vi "Read Summary.vi"(8 "error in (no error)":errorcluster, 11 "WfmAnalysator in":refnum<class "WfmAnalysator.lvclass">) -> (0 "error out":errorcluster, 1 "amplitude":dbl, 2 "period":dbl format="%.2g", 3 "WfmAnalysator out":refnum<class "WfmAnalysator.lvclass">)   [LabVIEW 2012, in "MyApp.lvlib" / "WfmAnalysator.lvclass"]
uses:
  WfmAnalysator.lvclass
  WfmAnalysator.lvclass/WfmAnalysator.ctl
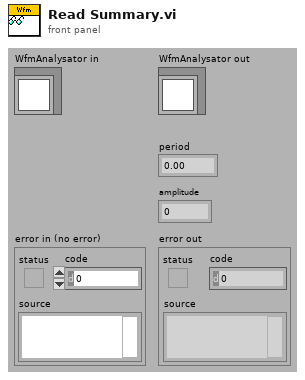
[diagram p1: front panel]
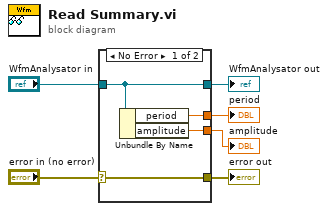
[diagram p0: block diagram]
diagram:
  n1 = case shown="No Error" "error in (no error)" {
    selector: "error in (no error)" -> [w10 w11]
    tunnel: [w10 w11] -> w5
    tunnel: [w9 w12] -> w3
    tunnel: "WfmAnalysator in" -> [w9 w12]
    tunnel: [w8 _] -> w2
    tunnel: [w7 _] -> w1
    frame No Error {
      n2 = Unbundle By Name(w9) -> ("period"=w8:dbl, "amplitude"=w7:dbl)
    }
    frame Error {
    }
  }
  "error out" <- w5
  "WfmAnalysator out" <- w3
  "period" <- w2
  "amplitude" <- w1
